vi "Parse Addr.vi"(8 "error in":errorcluster, 11 "Addr in":string) -> (0 "error out":errorcluster, 3 "Addr out":u16)   [LabVIEW 2018, in "Config Parser SPI_3W.lvlib" / "Config Parser SPI_3W.lvclass"]
uses:
  Config Parser SPI_3W.lvclass
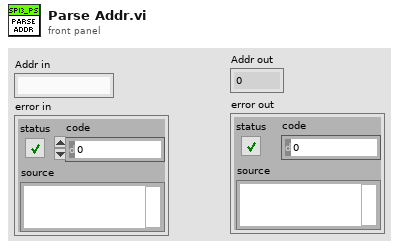
[diagram p1: front panel]
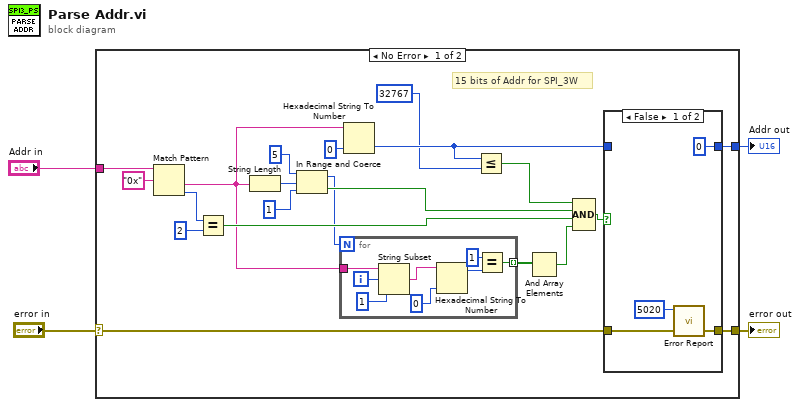
[diagram p0: block diagram]
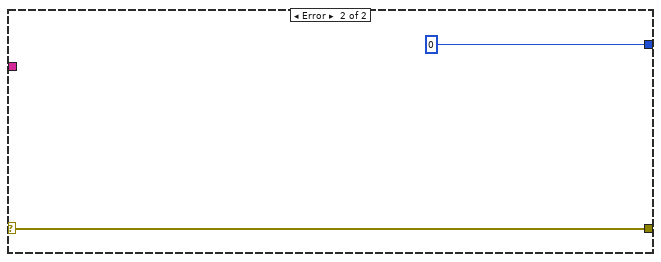
[diagram p3: hidden frame]
diagram:
  n1 = case shown="No Error" "error in" {
    selector: "error in" -> [w18 w41]
    tunnel: "Addr in" -> [w25 _]
    tunnel: [w17 w41] -> w1
    tunnel: [w16 u16 0] -> w2
    frame No Error {
      # "15 bits of Addr for SPI_3W"
      n2 = Match Pattern(string=w25, regular expression="0x") -> (after substring=w10:string, offset past match=w23:i32)  [unwired: 1 in, 2 out]
      n3 = Equal?(x=w23, y=2) -> (x = y?=w20:bool)
      n4 = String Length(string=w10) -> (length=w15:i32)
      n5 = In Range and Coerce(upper limit=5, x=w15, lower limit=1 ("upper limit")) -> (coerced(x)=w11:i32, In Range?=w12:bool)
      n6 = for {
        N: w11 -> [_]
        tunnel: w10 -> [w33]
        tunnel: [w26] -> w9 mode=indexing
        i -> [w32]
        n7 = String Subset(string=w33, offset (0)=w32, length (rest)=1 ("length (rest)")) -> (substring=w30:string)
        n8 = Hexadecimal String To Number(string=w30, default (0uL)=u16 0 ("Addr out")) -> (offset past number=w28:i32)  [unwired: 1 in, 1 out]
        n9 = Equal?(x=1, y=w28) -> (x = y?=w26:bool)
      }
      n10 = Hexadecimal String To Number(string=w10, default (0uL)=u16 0 ("Addr out")) -> (number=w7:u16)  [unwired: 1 in, 1 out]
      n11 = Less Or Equal?(x=w7, y=u16 32767) -> (x <= y?=w6:bool)
      n12 = And Array Elements(Boolean array=w9) -> (logical AND=w8:bool)
      n13 = Compound Arithmetic op=AND(w6, w12, w20, w8) -> (w19:bool)
      n14 = case shown="False" w19 {
        tunnel: w18 -> [w34 w39]
        tunnel: w7 -> [_ w38]
        tunnel: [w36 w39] -> w17
        tunnel: [u16 0 w38] -> w16
        frame False {
          n15 = call "Error Report.vi"("error in (no error)"=w34, "Error Code"=i16 5020) -> ("error out"=w36:errorcluster)  [unwired: 9 in]
        }
        frame True {
        }
      }
    }
    frame Error {
    }
  }
  "Addr out" <- w2
  "error out" <- w1
